vi "Calculate amplitude of array.vi"(11 "Array":dbl[](array[numeric])) -> (3 "A":dbl)   [LabVIEW 2020]
panel:
  # "Assuming sin wave like array, calculate amplitude A"
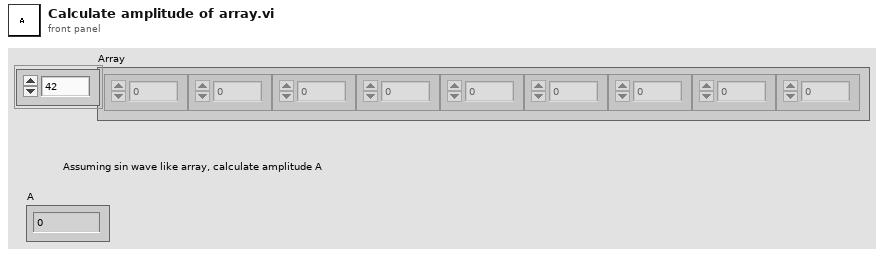
[diagram p1: front panel]
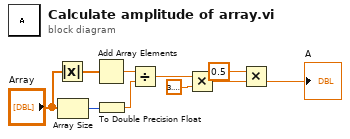
[diagram p0: block diagram]
diagram:
  n1 = Absolute Value(x="Array") -> (abs(x)=w10:dbl[])
  n2 = Array Size(array="Array") -> (size(s)=w7:i32)
  n3 = Add Array Elements(numeric array=w10) -> (sum=w9:dbl)
  n4 = To Double Precision Float(number=w7) -> (double precision float=w6:dbl)
  n5 = Divide(x=w9, y=w6) -> (x/y=w5:dbl)
  n6 = Multiply(x=w5, y=3.141592653589793) -> (x*y=w3:dbl)
  n7 = Multiply(x=0.5, y=w3) -> (x*y=→"A":dbl)
